vi "Configure Stream U6.vi"(1 "SettlingFactor":i32, 4 "Scan List (-)":u8[](array[numeric]), 6 "Wait Mode":string="LJ_swNONE", 7 "PC buffer size (seconds)":dbl=5.0 format="%.2f", 8 "error in":errorcluster, 9 "Scan List (+)":u8[](array[numeric])=[0, 1, 2, 3], 10 "Scan Rate (Hz)":dbl=1000.0 format="%.2f", 11 "Handle In":i32) -> (0 "error out":errorcluster, 2 "PC buffer size (samples)":i32=5, 3 "Handle Out":i32)   [LabVIEW 2021]
panel:
  # "The + scan list is the positive\nchannels.  For each element in\nthe + list, there must also be\nan element in the - list, which is\nthe negative channels.  For\nsingle-ended channels, put in\n199 for the negative channel."
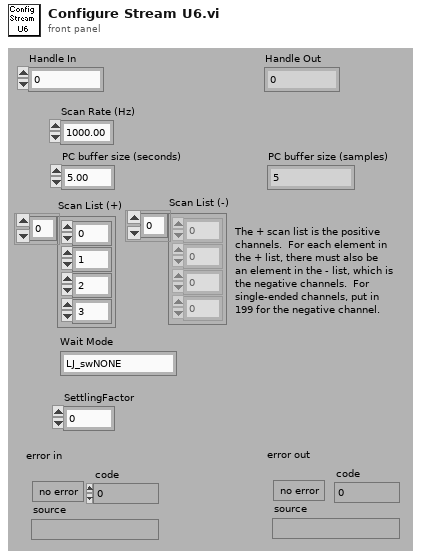
[diagram p1: front panel]
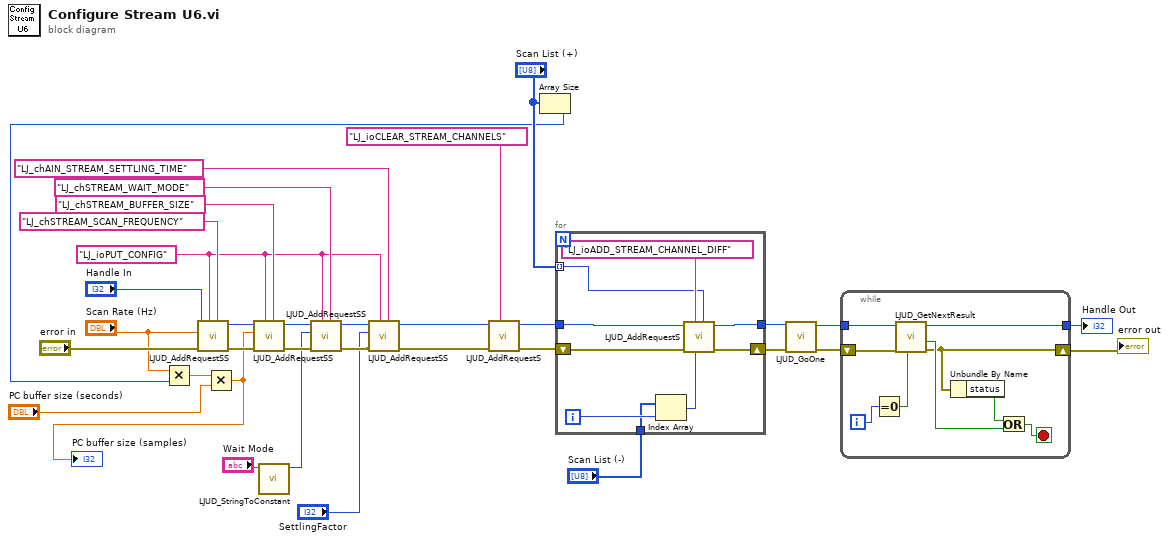
[diagram p0: block diagram]
diagram:
  w5 = "LJ_ioPUT_CONFIG" ("IOType")
  n1 = call "LJUD_AddRequestSS.vi"("Channel"="LJ_chSTREAM_SCAN_FREQUENCY" ("IOType"), "IOType"=w5, "error in"="error in", "Value"="Scan Rate (Hz)", "Handle In"="Handle In") -> ("error out"=w30:errorcluster, "Handle Out"=w32:i32)  [unwired: 5 in]
  n2 = call "LJUD_StringToConstant.vi"("String"="Wait Mode") -> ("Constant Number"=w12:i32)  [unwired: 9 in, 1 out]
  n3 = Array Size(array="Scan List (+)") -> (size(s)=w15:i32)
  n4 = Multiply(x="Scan Rate (Hz)", y=w15) -> (x*y=w20:dbl)
  n5 = Multiply(x=w20, y="PC buffer size (seconds)") -> (x*y=w9:dbl)
  "PC buffer size (samples)" <- w9
  n6 = call "LJUD_AddRequestSS.vi"("Channel"="LJ_chSTREAM_BUFFER_SIZE" ("IOType"), "IOType"=w5, "error in"=w30, "Value"=w9, "Handle In"=w32) -> ("error out"=w29:errorcluster, "Handle Out"=w31:i32)  [unwired: 5 in]
  n7 = call "LJUD_AddRequestSS.vi"("Channel"="LJ_chSTREAM_WAIT_MODE" ("IOType"), "IOType"=w5, "error in"=w29, "Value"=w12, "Handle In"=w31) -> ("error out"=w6:errorcluster, "Handle Out"=w7:i32)  [unwired: 5 in]
  n8 = call "LJUD_AddRequestSS.vi"("Channel"="LJ_chAIN_STREAM_SETTLING_TIME" ("IOType"), "IOType"=w5, "error in"=w6, "Value"="SettlingFactor", "Handle In"=w7) -> ("error out"=w3:errorcluster, "Handle Out"=w2:i32)  [unwired: 5 in]
  n9 = call "LJUD_AddRequestS.vi"("IOType"="LJ_ioCLEAR_STREAM_CHANNELS", "error in"=w3, "Handle In"=w2) -> ("error out"=w18:errorcluster, "Handle Out"=w19:i32)  [unwired: 7 in]
  n10 = for {
    tunnel: w19 -> [w43]
    shift-right: [w40] -> w24
    shift-left: w18 -> [w41]
    tunnel: "Scan List (+)" -> [w38] mode=indexing
    tunnel: [w39] -> w25
    tunnel: "Scan List (-)" -> [w36]
    i -> [w37]
    n11 = Index Array(array=w36, index=w37) -> (element=w35:u8)
    n12 = call "LJUD_AddRequestS.vi"("Channel"=w38, "x1"=w35, "IOType"="LJ_ioADD_STREAM_CHANNEL_DIFF", "error in"=w41, "Handle In"=w43) -> ("error out"=w40:errorcluster, "Handle Out"=w39:i32)  [unwired: 5 in]
  }
  n13 = call "LJUD_GoOne.vi"("error in"=w24, "Handle In"=w25) -> ("error out"=w11:errorcluster, "Handle Out"=w22:i32)  [unwired: 8 in]
  n14 = while {
    shift-left: w11 -> [w45]
    shift-right: [w44] -> w10
    tunnel: [w48] -> w23
    tunnel: w22 -> [w50]
    i -> [w47]
    stop <- w52 stop-if-true
    n15 = Equal To 0?(x=w47) -> (x = 0?=w51:bool)
    n16 = call "LJUD_GetNextResult.vi"("GetFirst"=w51, "error in"=w45, "Handle In"=w50) -> ("error out"=w44:errorcluster, "LJE_NO_MORE_DATA_AVAILABLE"=w46:bool, "Handle Out"=w48:i32)  [unwired: 3 in, 3 out]
    n17 = Unbundle By Name(w44) -> ("status"=w49:bool)
    n18 = Or(x=w49, y=w46) -> (x .or. y?=w52:bool)
  }
  "Handle Out" <- w23
  "error out" <- w10
